vi "Save TestStand ResultList to Excel AutoSearch.vi"(0 "Sequence Context":T1, 1 "Headers Path":path, 2 "report file path":path, 3 "start cell":cluster{"row":i32, "column":i32}, 5 "error in (no error)":errorcluster, 7 "WriteTheHeaders":bool) -> (17 "next cell":cluster{"row":i32, "column":i32}, 19 "error out":errorcluster)   [LabVIEW 2015]
doc: "This vi will search the array of column names for Column Name\nand save an array of results starting at the point where Column Name is found\nBe sure to copy the name of the first Step with a result to the Column Name input"
uses:
  <vilib>/addons/TestStand/_TSLegacy.llb/LabVIEW Test - Sequence Context.ctl
  <vilib>/addons/TestStand/_TSUtility.llb/TestStand - Get Property Value (String Array).vi
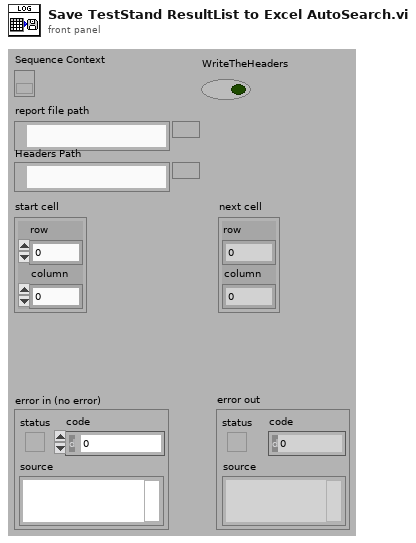
[diagram p1: front panel]
types:
  T1 = typedef "LabVIEW Test - Sequence Context.ctl" = refnum<k7>
  T2 = typedef "Test Result.ctl" = cluster{"StepName":string, "Status":bool, "Data":string, "Limits":variant}
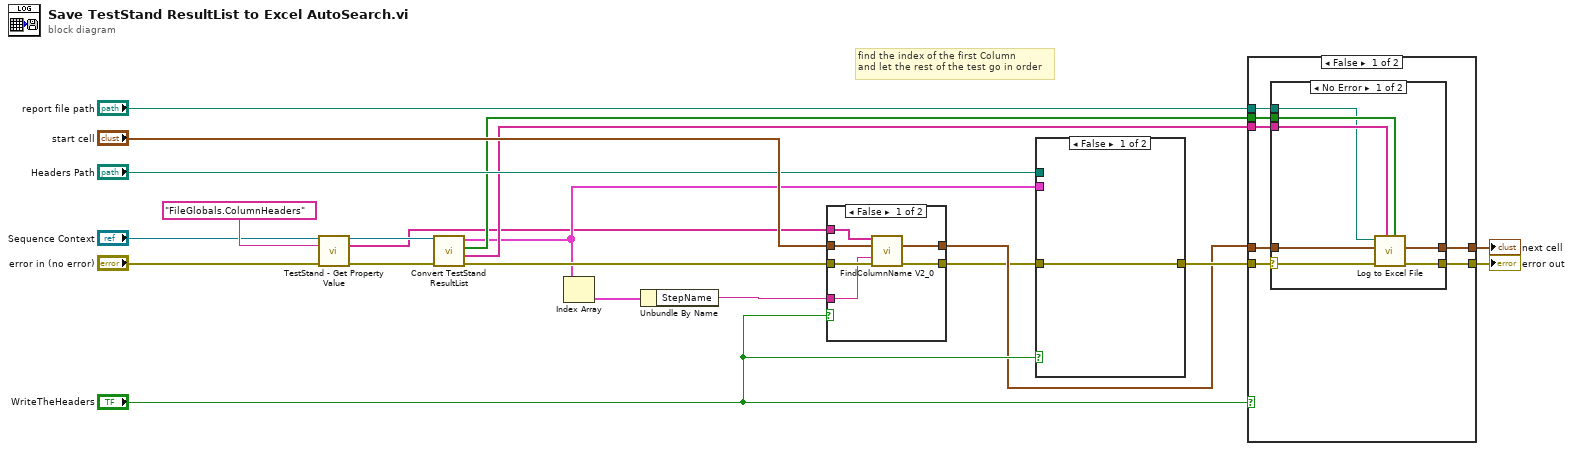
[diagram p0: block diagram]
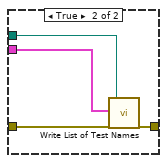
[diagram p5: hidden frame]
diagram:
  # "find the index of the first Column\nand let the rest of the test go in order"
  n1 = call-poly <vilib>:"TestStand - Get Property Value.vi"("Sequence Context In"="Sequence Context", "Lookup String"="FileGlobals.ColumnHeaders", "error in (no error)"="error in (no error)") -> ("Sequence Context Out"=w4:refnum<k7>, "Value"=w1:string[], "error out"=w2:errorcluster)  [unwired: 10 in]
  n2 = call "Convert TestStand ResultList.vi"("error in (no error)"=w2, "Sequence Context"=w4) -> ("error out"=w11:errorcluster, "data"=w12:string[], "status"=w15:bool[], "Results"=w9:T2[])  [unwired: 6 in]
  n3 = Index Array(array=w9) -> (element=w8:T2)  [unwired: 1 in]
  n4 = Unbundle By Name(w8) -> ("StepName"=w7:string)
  n5 = case shown="False" "WriteTheHeaders" {
    tunnel: w11 -> [w27 w28]
    tunnel: [w26 w28] -> w10
    tunnel: "start cell" -> [w25 w29]
    tunnel: [w24 w29] -> w13
    tunnel: w7 -> [w23 _]
    tunnel: w1 -> [w22 _]
    frame False {
      n6 = call "FindColumnName V2_0.vi"("Columns"=w22, "start cell in"=w25, "Column Name"=w23, "error in (no error)"=w27) -> ("start cell out"=w24:cluster{"row":i32, "column":i32}, "error out"=w26:errorcluster)  [unwired: 10 in]
    }
    frame True {
    }
  }
  n7 = case shown="False" "WriteTheHeaders" {
    tunnel: w10 -> [w30 w34]
    tunnel: [w30 w33] -> w14
    tunnel: w9 -> [_ w32]
    tunnel: "Headers Path" -> [_ w31]
    frame False {
    }
    frame True {
      n8 = call "Write List of Test Names.vi"("Results"=w32, "error in (no error)"=w34, "file path (use dialog)"=w31) -> ("error out"=w33:errorcluster)  [unwired: 16 in]
    }
  }
  n9 = case shown="False" "WriteTheHeaders" {
    tunnel: w15 -> [w41 _]
    tunnel: [w40 w52] -> w21
    tunnel: "report file path" -> [w39 _]
    tunnel: [w38 w51] -> w19
    tunnel: w14 -> [w37 w52]
    tunnel: w13 -> [w36 w51]
    tunnel: w12 -> [w35 _]
    frame False {
      n10 = case shown="No Error" w37 {
        selector: w37 -> [w42 w50]
        tunnel: w41 -> [w48 _]
        tunnel: w35 -> [w47 _]
        tunnel: [w46 w50] -> w40
        tunnel: w39 -> [w45 _]
        tunnel: w36 -> [w43 w49]
        tunnel: [w44 w49] -> w38
        frame No Error {
          n11 = call "Log to Excel File.vi"("status"=w48, "data"=w47, "error in"=w42, "start cell"=w43, "report file path"=w45) -> ("error out"=w46:errorcluster, "next cell"=w44:cluster{"row":i32, "column":i32})  [unwired: 5 in]
        }
        frame Error {
        }
      }
    }
    frame True {
    }
  }
  "error out" <- w21
  "next cell" <- w19
